vi "Temp.Simple State Machine.vi"(8 "Error In":errorcluster) -> (0 "Error Out":errorcluster)   [LabVIEW 2018]
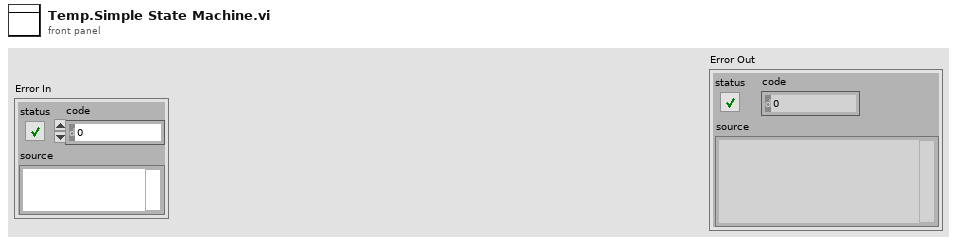
[diagram p1: front panel]
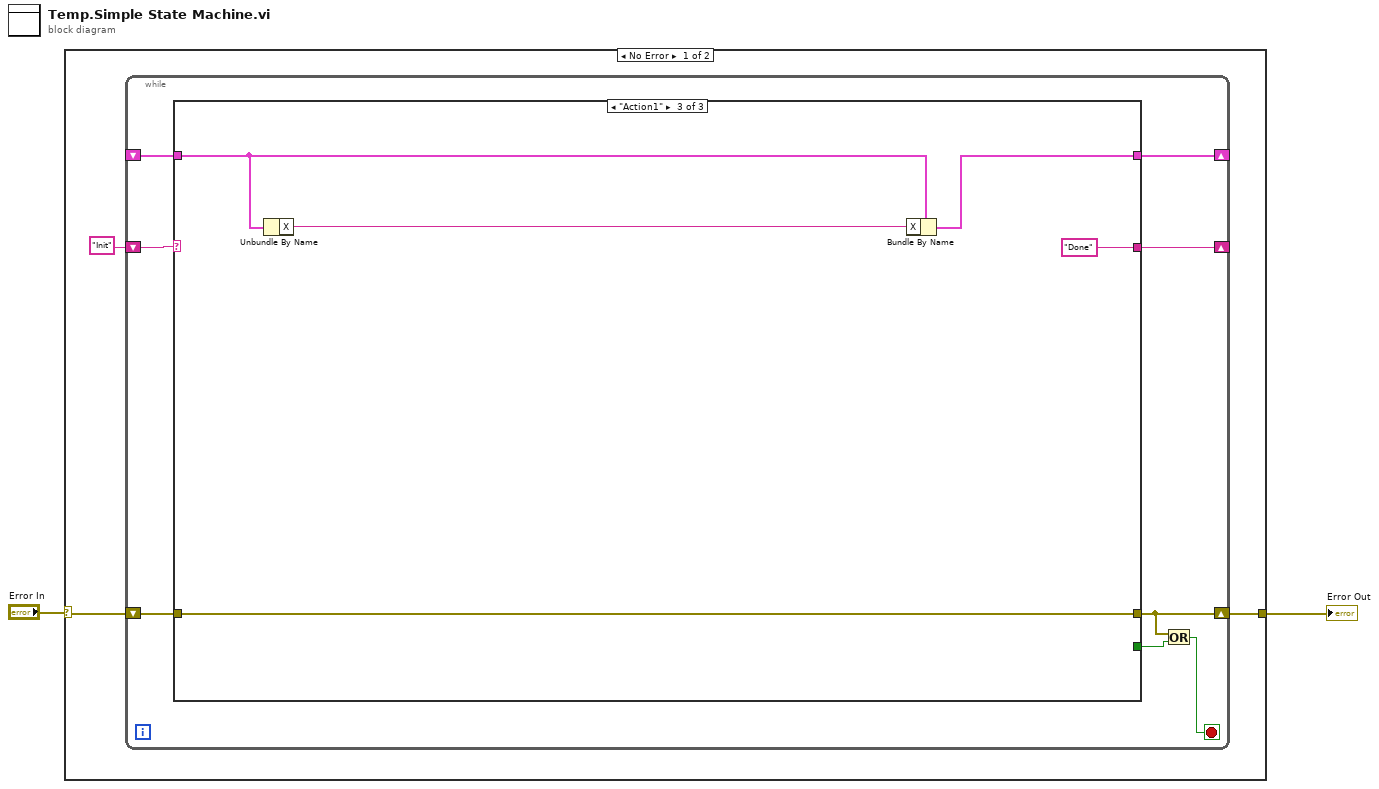
[diagram p0: block diagram]
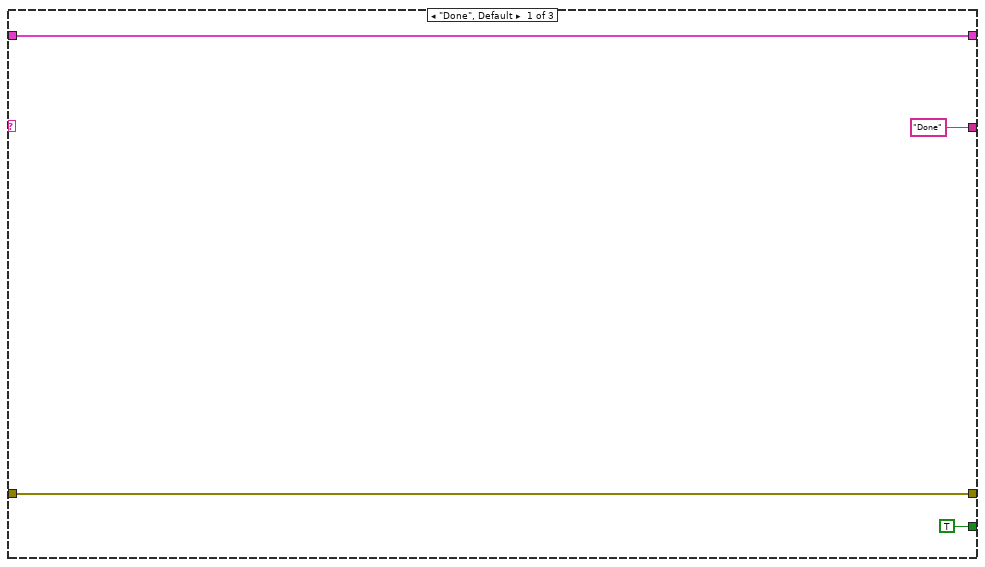
[diagram p2: hidden frame]
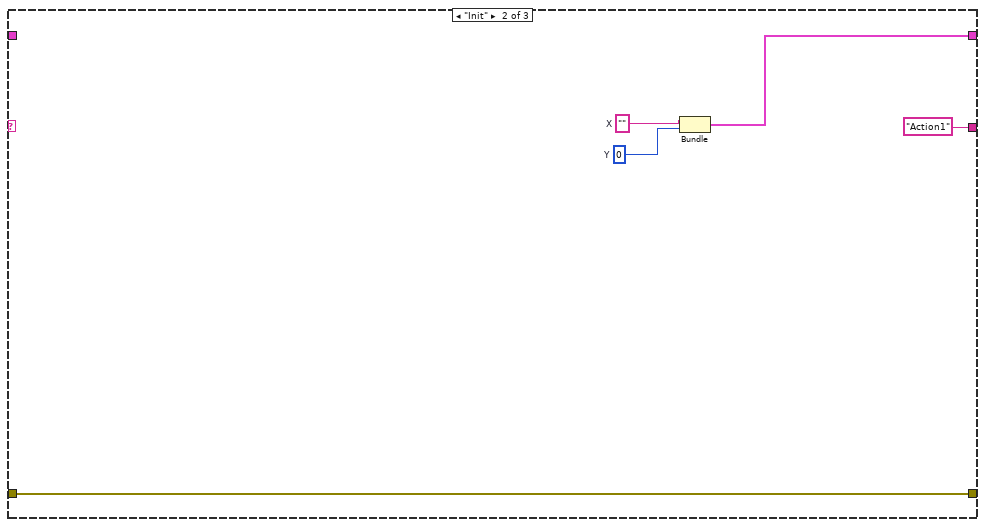
[diagram p3: hidden frame]
diagram:
  n1 = case shown="No Error" "Error In" {
    selector: "Error In" -> [w3 w28]
    tunnel: [w4 w28] -> w2
    frame No Error {
      n2 = while {
        shift-right: [w8] -> _
        shift-left: _ -> [w13]
        shift-right: [w7] -> _
        shift-left: "Init" -> [w9]
        shift-right: [w11] -> w4
        shift-left: w3 -> [w12]
        stop <- w10 stop-if-true
        n3 = case shown="\"Action1\"" w9 {
          tunnel: w13 -> [w17 _ w25]
          tunnel: w12 -> [w15 w22 w26]
          tunnel: [w15 w22 w26] -> w11
          tunnel: [w17 w19 w24] -> w8
          tunnel: ["Done" "Action1" "Done"] -> w7
          tunnel: [TRUE _ _] -> w6
          frame "Done", Default {
          }
          frame "Init" {
            w20 = 0  # Y
            w21 = ""  # X
            n4 = Bundle("X"=w21, "Y"=w20) -> (w19:cluster{"X":string, "Y":i32})  [unwired: 1 in]
          }
          frame "Action1" {
            n5 = Unbundle By Name(w25) -> ("X"=w23:string)
            n6 = Bundle By Name(cluster=w25, "X"=w23) -> (w24:cluster{"X":string, "Y":i32})
          }
        }
        n7 = Or(x=w11, y=w6) -> (x .or. y?=w10:bool)
      }
    }
    frame Error {
    }
  }
  "Error Out" <- w2
